vi "SquareRootBrianSheridan.vi"() -> ()   [LabVIEW 2014]
panel:
  out "Square Root Value":dbl
  in  "Numeric":dbl
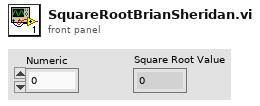
[diagram p1: front panel]
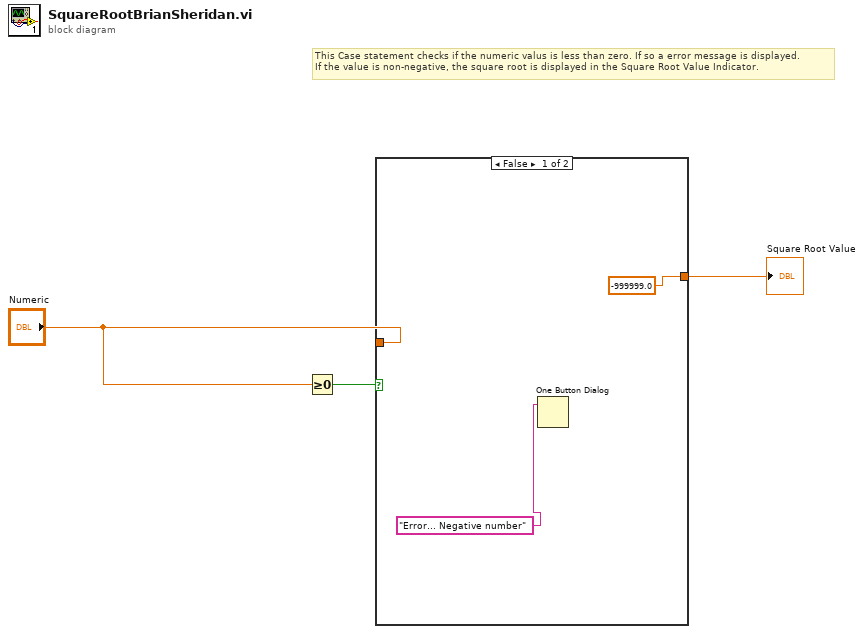
[diagram p0: block diagram]
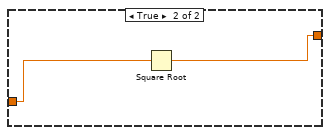
[diagram p2: hidden frame]
diagram:
  # "This Case statement checks if the numeric valus is less than zero. If so a error message is displayed.\nIf the value is non-negative, the square root is displayed in the Square Root Value Indicator."
  n1 = Greater Or Equal To 0?(x="Numeric") -> (x >= 0?=w2:bool)
  n2 = case shown="False" w2 {
    tunnel: [-999999.0 w7] -> w3
    tunnel: "Numeric" -> [_ w6]
    frame False {
      n3 = One Button Dialog(message="Error... Negative number" ("button name (\"OK\")")) -> ()  [unwired: 1 in, 1 out]
    }
    frame True {
      n4 = Square Root(x=w6) -> (sqrt(x)=w7:dbl)
    }
  }
  "Square Root Value" <- w3
